vi "Open.vi"(7 "Allow multiple opens?":bool, 8 "error in (no error)":errorcluster, 10 "Channel Name":tag) -> (0 "error out":errorcluster, 3 "I2C Ref Out":T1={"myRIO Reference"={"myRIO Model"=enum."Unknown", "myRIO Hardware Reference"={"Generic FPGA Reference"=refnum, "Allow multiple opens"=FALSE}}, "I2C Channels Enum"=enum."Not Connected", "I2C Configuration"={"I2C Transfer Rate"=enum."Fast mode (400 kbps)"}})   [LabVIEW 2021, in "I2C.lvlib"]
doc: "Opens a reference to an Inter-Integrated Circuit (I2C) channel. You must open a reference before you use an I2C channel to write/read data to/from an I2C slave device."
uses:
  <vilib>/myRIO/Instrument Drivers/Onboard IO/I2C/I2C.lvlib
  <vilib>/myRIO/Instrument Drivers/Onboard IO/I2C/typedefs/I2C Reference.ctl
  <vilib>/myRIO/Common/Instrument Driver Framework/Utilities/typedefs/myRIO Generic Hardware Reference.ctl
  <vilib>/myRIO/Common/Instrument Driver Framework/Utilities/typedefs/Hardware Version Enum.ctl
  <vilib>/myRIO/Common/Instrument Driver Framework/Utilities/typedefs/myRIO v1.0 Reference.ctl
  <vilib>/myRIO/Common/Instrument Driver Framework/Utilities/typedefs/Generic FPGA Reference.ctl
  <vilib>/myRIO/Common/Instrument Driver Framework/myRIO v1.0/I2C/typedefs/I2C Channels Enum.ctl
  <vilib>/myRIO/Instrument Drivers/Onboard IO/I2C/typedefs/I2C Configuration.ctl
  <vilib>/myRIO/Instrument Drivers/Onboard IO/I2C/typedefs/I2C Transfer Rate.ctl
  <vilib>/myRIO/Common/Instrument Driver Framework/Utilities/vis/Validate Channels.vi
  <vilib>/myRIO/Common/Instrument Driver Framework/myRIO v1.0/I2C/vis/myRIO v1.0 Reserve I2C.vi
  <vilib>/myRIO/Common/Instrument Driver Framework/roboRIO v1.0/I2C/vis/roboRIO v1.0 Reserve I2C.vi
  <vilib>/myRIO/Common/Instrument Driver Framework/ELVIS III v1.0/I2C/vis/ELVIS III v1.0 Reserve I2C.vi
  <vilib>/myRIO/Common/Instrument Driver Framework/myRIO v1.0/I2C/vis/myRIO v1.0 Build MUX Configuration I2C.vi
  <vilib>/myRIO/Common/Instrument Driver Framework/myRIO v1.0/Resource Manager/vis/myRIO v1.0 Reserve Channel List.vi
  <vilib>/myRIO/Common/Instrument Driver Framework/roboRIO v1.0/Resource Manager/vis/roboRIO v1.0 Reserve Channel List.vi
  <vilib>/myRIO/Common/Instrument Driver Framework/roboRIO v1.0/I2C/vis/roboRIO v1.0 Build MUX Configuration I2C.vi
  <vilib>/myRIO/Common/Instrument Driver Framework/ELVIS III v1.0/I2C/vis/ELVIS III v1.0 Build MUX Configuration I2C.vi
  <vilib>/myRIO/Common/Instrument Driver Framework/myRIO v1.0/Resource Manager/vis/myRIO v1.0 Create Configuration List.vi
  <vilib>/myRIO/Common/Instrument Driver Framework/myRIO v1.0/Resource Manager/vis/myRIO v1.0 Reserve Channel.vi
  <vilib>/myRIO/Common/Instrument Driver Framework/myRIO v1.0/Resource Manager/vis/myRIO v1.0 Unreserve Channel.vi
  <vilib>/myRIO/Common/Instrument Driver Framework/roboRIO v1.0/Resource Manager/vis/roboRIO v1.0 Reserve Channel.vi
  <vilib>/myRIO/Common/Instrument Driver Framework/roboRIO v1.0/Resource Manager/vis/roboRIO v1.0 Unreserve Channel.vi
  <vilib>/myRIO/Common/Instrument Driver Framework/roboRIO v1.0/Resource Manager/vis/roboRIO v1.0 Create Configuration List.vi
  <vilib>/myRIO/Common/Instrument Driver Framework/ELVIS III v1.0/Resource Manager/vis/ELVIS III v1.0 Create Configuration List.vi
  <vilib>/myRIO/Common/Instrument Driver Framework/myRIO v1.0/Resource Manager/vis/myRIO v1.0 Build Mutex Name.vi
  <vilib>/myRIO/Common/Instrument Driver Framework/roboRIO v1.0/Resource Manager/vis/roboRIO v1.0 Build Mutex Name.vi
  <vilib>/Utility/VariantDataType/GetNumericInfo.vi
  <vilib>/myRIO/Common/Instrument Driver Framework/Utilities/vis/IO Manager.vi
  <vilib>/myRIO/Common/Instrument Driver Framework/Utilities/vis/Configuration Manager.vi
  <vilib>/myRIO/Common/Instrument Driver Framework/myRIO v1.0/Resource Manager/vis/myRIO v1.0 Configure IO.vi
  <vilib>/myRIO/Common/Instrument Driver Framework/myRIO v1.0/myRIO v1.0 Close.vi
  <vilib>/myRIO/Common/Instrument Driver Framework/roboRIO v1.0/Resource Manager/vis/roboRIO v1.0 Configure IO.vi
  <vilib>/myRIO/Common/Instrument Driver Framework/ELVIS III v1.0/Resource Manager/vis/ELVIS III v1.0 Reserve Channel List.vi
  <vilib>/myRIO/Common/Instrument Driver Framework/ELVIS III v1.0/Resource Manager/vis/ELVIS III v1.0 Configure IO.vi
  <vilib>/userdefined/High Color/nirio_resource_hc.ctl
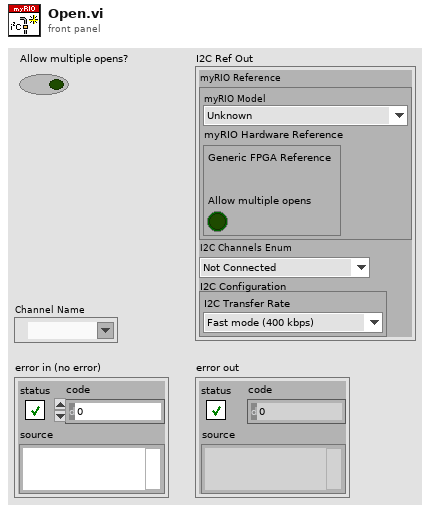
[diagram p1: front panel]
types:
  T1 = typedef "I2C.lvlib/I2C Reference.ctl" = cluster{"myRIO Reference":T2, "I2C Channels Enum":T6, "I2C Configuration":T7}
  T2 = typedef "myRIO Generic Hardware Reference.ctl" = cluster{"myRIO Model":T3, "myRIO Hardware Reference":T4}
  T3 = typedef "Hardware Version Enum.ctl" = enum16{"Unknown", "myRIO-1900", "myRIO-1950", "roboRIO", "NI ELVIS RIO CM", "ELVIS III"}
  T4 = typedef "myRIO v1.0 Reference.ctl" = cluster{"Generic FPGA Reference":T5, "Allow multiple opens":bool}
  T5 = typedef "Generic FPGA Reference.ctl" = refnum<k20>
  T6 = typedef "I2C Channels Enum.ctl" = enum16{"Not Connected", "A/I2C", "B/I2C", "I2C/I2C"}
  T7 = typedef "I2C.lvlib/I2C Configuration.ctl" = cluster{"I2C Transfer Rate":T8}
  T8 = typedef "I2C.lvlib/I2C Transfer Rate.ctl" = enum16{"Standard mode (100 kbps)", "Fast mode (400 kbps)"}
  T9 = typedef "nirio_resource_hc.ctl" = tag
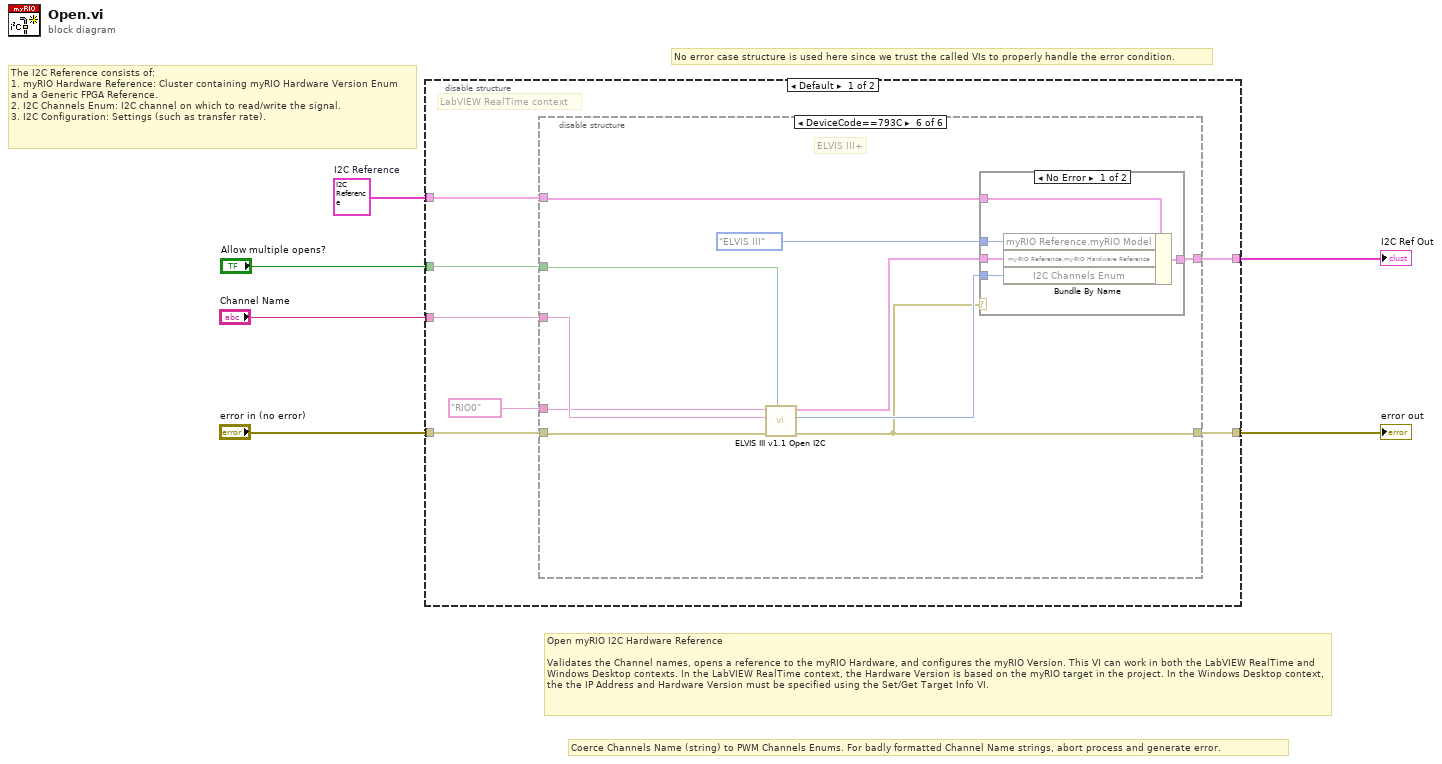
[diagram p0: block diagram]
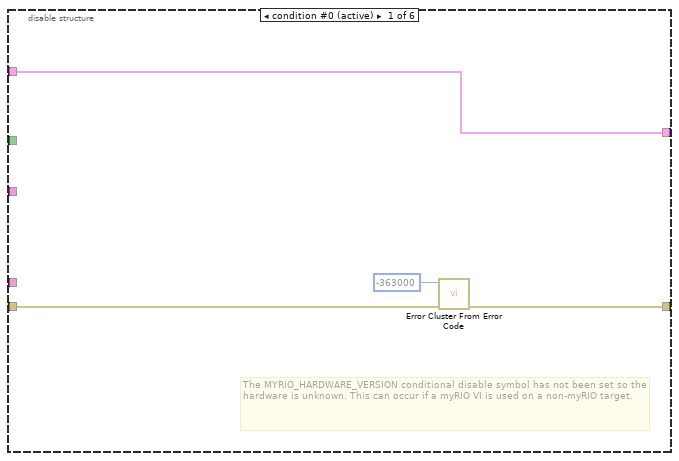
[diagram p2: hidden frame]
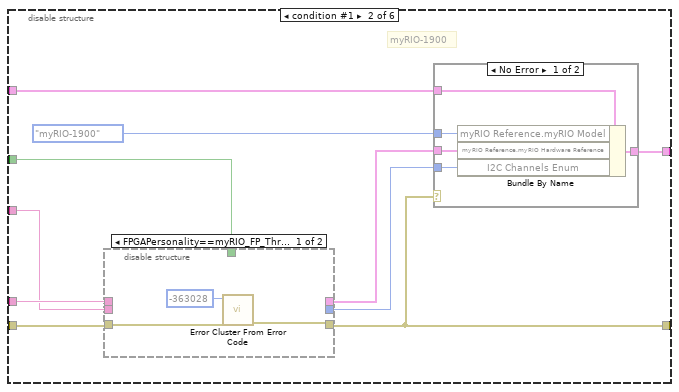
[diagram p3: hidden frame]
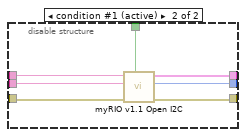
[diagram p4: hidden frame]
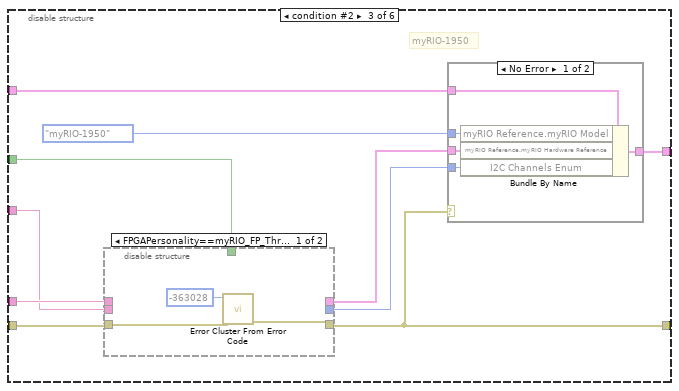
[diagram p6: hidden frame]
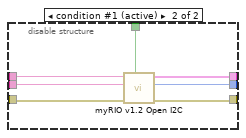
[diagram p7: hidden frame]
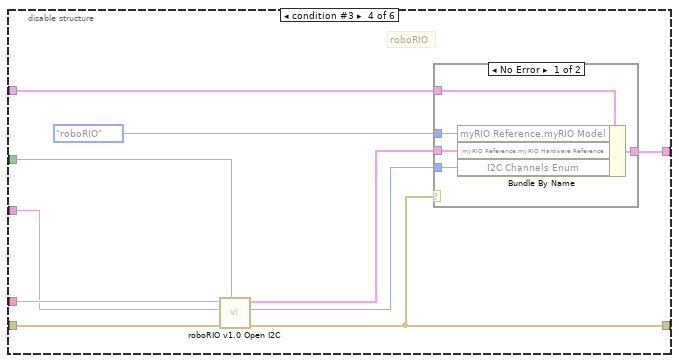
[diagram p9: hidden frame]
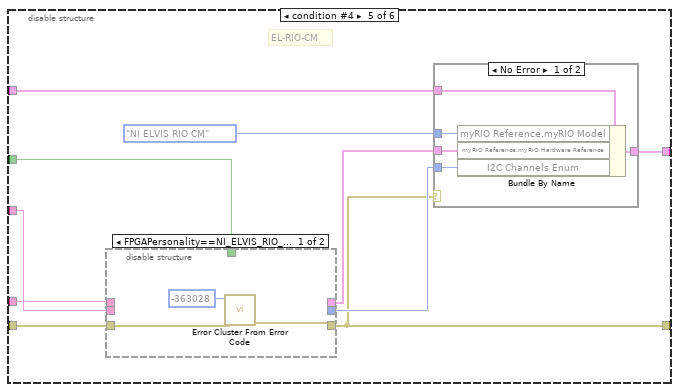
[diagram p11: hidden frame]
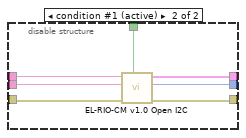
[diagram p12: hidden frame]
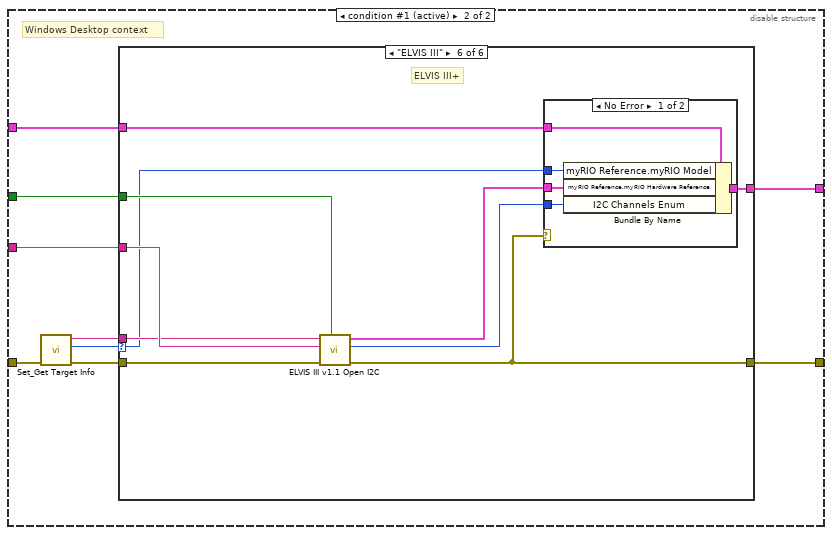
[diagram p15: hidden frame]
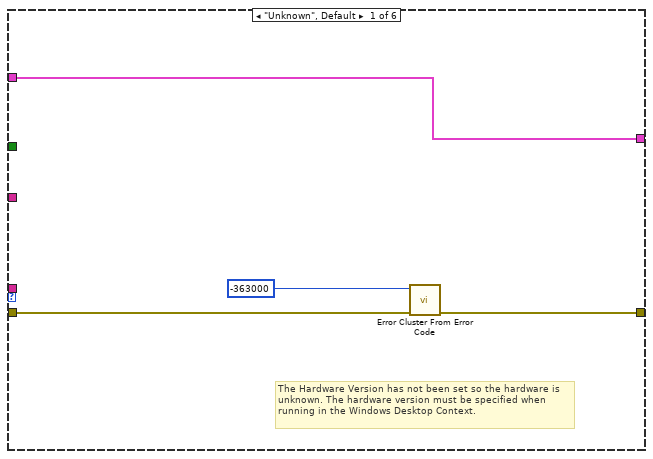
[diagram p16: hidden frame]
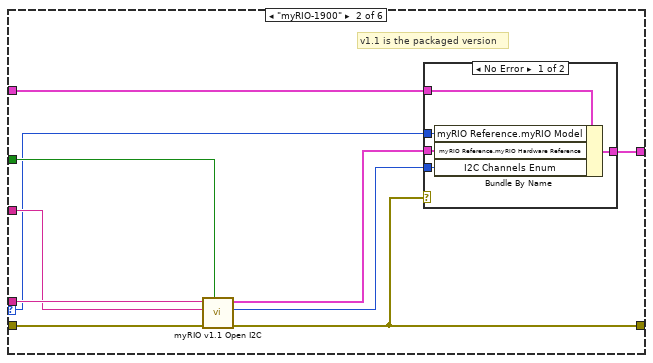
[diagram p17: hidden frame]
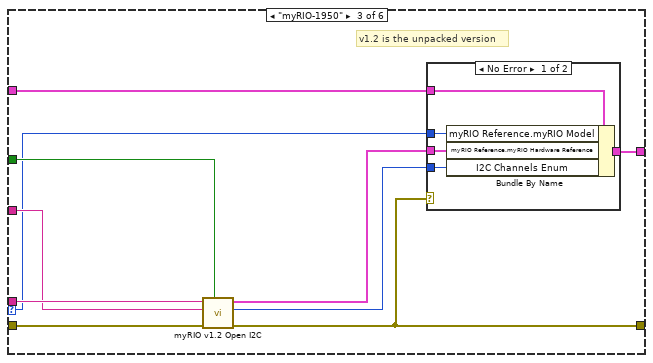
[diagram p19: hidden frame]
diagram:
  w6 = T1 {"myRIO Reference"={"myRIO Model"=enum."Unknown", "myRIO Hardware Reference"={"Generic FPGA Reference"=refnum, "Allow multiple opens"=FALSE}}, "I2C Channels Enum"=enum."Not Connected", "I2C Configuration"={"I2C Transfer Rate"=enum."Standard mode (100 kbps)"}}  # I2C Reference
  # "No error case structure is used here since we trust the called VIs to properly handle the error condition."
  # "Open myRIO I2C Hardware Reference\n\nValidates the Channel names, opens a reference to the myRIO Hardware, and configures the myRIO Version. This VI can work in both the LabVIEW RealTime and Windows Desktop contexts. In the LabVIEW RealTime context, the Hardware Version is based on the myRIO target in the project. In the Windows Desktop context, the the IP Address and Hardware Version must be specified using the Set/Get Target Info VI."
  # "The I2C Reference consists of:\n1. myRIO Hardware Reference: Cluster containing myRIO Hardware Version Enum and a Generic FPGA Reference.\n2. I2C Channels Enum: I2C channel on which to read/write the signal.\n3. I2C Configuration: Settings (such as transfer rate)."
  # "Coerce Channels Name (string) to PWM Channels Enums. For badly formatted Channel Name strings, abort process and generate error."
  n1 = disable-structure shown="Default" {
    disable-tunnel: [w13 w136] -> w4
    disable-tunnel: "error in (no error)" -> [w12 w133]
    disable-tunnel: [w11 w135] -> w3
    disable-tunnel: w6 -> [w10 w134]
    disable-tunnel: "Channel Name" -> [w8 w129]
    disable-tunnel: "Allow multiple opens?" -> [w7 w128]
    frame condition #0 {
      # "LabVIEW RealTime context"
      n2 = disable-structure shown="DeviceCode==793C" {
        disable-tunnel: [w16 w18 w44 w70 w87 w113] -> w13
        disable-tunnel: [w14 w24 w50 w76 w94 w112] -> w11
        disable-tunnel: w12 -> [w15 w25 w51 w77 w92 w114]
        disable-tunnel: w10 -> [w14 w23 w49 w75 w93 w118]
        disable-tunnel: T9 "RIO0" ("resource name") -> [_ w22 w48 w74 w90 w115]
        disable-tunnel: w8 -> [_ w21 w47 w73 w91 w116]
        disable-tunnel: w7 -> [_ w19 w45 w71 w86 w117]
        frame condition #0 (active) {
          # "The MYRIO_HARDWARE_VERSION conditional disable symbol has not been set so the hardware is unknown. This can occur if a myRIO VI is used on a non-myRIO target."
          n3 = call <vilib>:"Error Cluster From Error Code.vi"("error in (no error)"=w15, "error code (0)"=-363000) -> ("error out"=w16:errorcluster)  [unwired: 7 in]
        }
        frame condition #1 {
          # "myRIO-1900"
          n4 = disable-structure shown="FPGAPersonality==myRIO_FP_Throughput" {
            disable-tunnel: [_ w37] -> w26
            disable-tunnel: w25 -> [w29 w36]
            disable-tunnel: w22 -> [_ w35]
            disable-tunnel: w21 -> [_ w34]
            disable-tunnel: [_ w33] -> w20
            disable-tunnel: w19 -> [_ w32]
            disable-tunnel: [w28 w31] -> w18
            frame condition #0 {
              n5 = call <vilib>:"Error Cluster From Error Code.vi"("error in (no error)"=w29, "error code (0)"=-363028) -> ("error out"=w28:errorcluster)  [unwired: 7 in]
            }
            frame condition #1 (active) {
              n6 = call <vilib>:"myRIO v1.1 Open I2C.vi"("Allow multiple opens?"=w32, "error in (no error)"=w36, "Channel Name"=w34, "Resource name"=w35) -> ("error out"=w31:errorcluster, "I2C Channel"=w33:T6, "myRIO Ref Out"=w37:T4)  [unwired: 5 in]
            }
          }
          n7 = case shown="No Error" w18 {
            tunnel: Hardware_Version_Enum."myRIO-1900" ("Hardware Version") -> [w42 _]
            tunnel: w26 -> [w41 _]
            tunnel: [w40 w43] -> w24
            tunnel: w23 -> [w39 w43]
            tunnel: w20 -> [w38 _]
            frame No Error {
              n8 = Bundle By Name(cluster=w39, "myRIO Reference.myRIO Model"=w42, "myRIO Reference.myRIO Hardware Reference"=w41, "I2C Channels Enum"=w38) -> (w40:T1)
            }
            frame Error {
            }
          }
        }
        frame condition #2 {
          # "myRIO-1950"
          n9 = disable-structure shown="FPGAPersonality==myRIO_FP_Throughput" {
            disable-tunnel: [_ w63] -> w52
            disable-tunnel: w51 -> [w55 w62]
            disable-tunnel: w48 -> [_ w61]
            disable-tunnel: w47 -> [_ w60]
            disable-tunnel: [_ w59] -> w46
            disable-tunnel: w45 -> [_ w58]
            disable-tunnel: [w54 w57] -> w44
            frame condition #0 {
              n10 = call <vilib>:"Error Cluster From Error Code.vi"("error in (no error)"=w55, "error code (0)"=-363028) -> ("error out"=w54:errorcluster)  [unwired: 7 in]
            }
            frame condition #1 (active) {
              n11 = call <vilib>:"myRIO v1.2 Open I2C.vi"("Allow multiple opens?"=w58, "error in (no error)"=w62, "Channel Name"=w60, "Resource name"=w61) -> ("error out"=w57:errorcluster, "I2C Channel"=w59:T6, "myRIO Ref Out"=w63:T4)  [unwired: 5 in]
            }
          }
          n12 = case shown="No Error" w44 {
            tunnel: Hardware_Version_Enum."myRIO-1950" ("Hardware Version") -> [w68 _]
            tunnel: w52 -> [w67 _]
            tunnel: [w66 w69] -> w50
            tunnel: w49 -> [w65 w69]
            tunnel: w46 -> [w64 _]
            frame No Error {
              n13 = Bundle By Name(cluster=w65, "myRIO Reference.myRIO Model"=w68, "myRIO Reference.myRIO Hardware Reference"=w67, "I2C Channels Enum"=w64) -> (w66:T1)
            }
            frame Error {
            }
          }
        }
        frame condition #3 {
          # "roboRIO"
          n14 = call <vilib>:"roboRIO v1.0 Open I2C.vi"("Allow multiple opens?"=w71, "error in (no error)"=w77, "Channel Name"=w73, "Resource name"=w74) -> ("error out"=w70:errorcluster, "I2C Channel"=w72:T6, "myRIO Ref Out"=w78:T4)  [unwired: 5 in]
          n15 = case shown="No Error" w70 {
            tunnel: Hardware_Version_Enum."roboRIO" ("Hardware Version") -> [w84 _]
            tunnel: w78 -> [w83 _]
            tunnel: [w82 w85] -> w76
            tunnel: w75 -> [w81 w85]
            tunnel: w72 -> [w80 _]
            frame No Error {
              n16 = Bundle By Name(cluster=w81, "myRIO Reference.myRIO Model"=w84, "myRIO Reference.myRIO Hardware Reference"=w83, "I2C Channels Enum"=w80) -> (w82:T1)
            }
            frame Error {
            }
          }
        }
        frame condition #4 {
          # "EL-RIO-CM"
          n17 = disable-structure shown="FPGAPersonality==NI_ELVIS_RIO_CM_FP_Throughput" {
            disable-tunnel: [_ w105] -> w89
            disable-tunnel: w92 -> [w97 w100]
            disable-tunnel: w90 -> [_ w102]
            disable-tunnel: w91 -> [_ w101]
            disable-tunnel: [_ w104] -> w88
            disable-tunnel: w86 -> [_ w99]
            disable-tunnel: [w96 w103] -> w87
            frame condition #0 {
              n18 = call <vilib>:"Error Cluster From Error Code.vi"("error in (no error)"=w97, "error code (0)"=-363028) -> ("error out"=w96:errorcluster)  [unwired: 7 in]
            }
            frame condition #1 (active) {
              n19 = call <vilib>:"EL-RIO-CM v1.0 Open I2C.vi"("Allow multiple opens?"=w99, "error in (no error)"=w100, "Channel Name"=w101, "Resource name"=w102) -> ("error out"=w103:errorcluster, "I2C Channel"=w104:T6, "myRIO Ref Out"=w105:T4)  [unwired: 5 in]
            }
          }
          n20 = case shown="No Error" w87 {
            tunnel: Hardware_Version_Enum."NI ELVIS RIO CM" ("Hardware Version") -> [w110 _]
            tunnel: w89 -> [w109 _]
            tunnel: [w108 w111] -> w94
            tunnel: w93 -> [w107 w111]
            tunnel: w88 -> [w106 _]
            frame No Error {
              n21 = Bundle By Name(cluster=w107, "myRIO Reference.myRIO Model"=w110, "myRIO Reference.myRIO Hardware Reference"=w109, "I2C Channels Enum"=w106) -> (w108:T1)
            }
            frame Error {
            }
          }
        }
        frame condition #5 {
          # "ELVIS III+"
          n22 = call <vilib>:"ELVIS III v1.1 Open I2C.vi"("Allow multiple opens?"=w117, "error in (no error)"=w114, "Channel Name"=w116, "Resource name"=w115) -> ("error out"=w113:errorcluster, "I2C Channel"=w119:T6, "myRIO Ref Out"=w120:T4)  [unwired: 5 in]
          n23 = case shown="No Error" w113 {
            tunnel: Hardware_Version_Enum."ELVIS III" ("Hardware Version") -> [w126 _]
            tunnel: w120 -> [w125 _]
            tunnel: [w124 w127] -> w112
            tunnel: w118 -> [w123 w127]
            tunnel: w119 -> [w122 _]
            frame No Error {
              n24 = Bundle By Name(cluster=w123, "myRIO Reference.myRIO Model"=w126, "myRIO Reference.myRIO Hardware Reference"=w125, "I2C Channels Enum"=w122) -> (w124:T1)
            }
            frame Error {
            }
          }
        }
      }
    }
    frame condition #1 (active) {
      # "Windows Desktop context"
      n25 = call <vilib>:"Set_Get Target Info.vi"("error in (no error)"=w133) -> ("error out"=w132:errorcluster, "Hardware Version"=w131:T3, "IP Address"=w130:string)  [unwired: 8 in]
      n26 = case shown="\"ELVIS III\"" w131 {
        selector: w131 -> [_ w141 w157 w173 w189 w208]
        tunnel: [w139 w142 w158 w174 w190 w206] -> w136
        tunnel: w132 -> [w138 w147 w163 w179 w195 w207]
        tunnel: [w137 w149 w165 w181 w197 w205] -> w135
        tunnel: w134 -> [w137 w148 w164 w180 w196 w212]
        tunnel: w130 -> [_ w146 w162 w178 w194 w209]
        tunnel: w129 -> [_ w145 w161 w177 w193 w210]
        tunnel: w128 -> [_ w143 w159 w175 w191 w211]
        frame "Unknown", Default {
          # "The Hardware Version has not been set so the hardware is unknown. The hardware version must be specified when running in the Windows Desktop Context."
          n27 = call <vilib>:"Error Cluster From Error Code.vi"("error in (no error)"=w138, "error code (0)"=-363000) -> ("error out"=w139:errorcluster)  [unwired: 7 in]
        }
        frame "myRIO-1900" {
          # "v1.1 is the packaged version"
          n28 = call <vilib>:"myRIO v1.1 Open I2C.vi"("Allow multiple opens?"=w143, "error in (no error)"=w147, "Channel Name"=w145, "Resource name"=w146) -> ("error out"=w142:errorcluster, "I2C Channel"=w144:T6, "myRIO Ref Out"=w150:T4)  [unwired: 5 in]
          n29 = case shown="No Error" w142 {
            tunnel: w141 -> [w155 _]
            tunnel: w150 -> [w154 _]
            tunnel: [w153 w156] -> w149
            tunnel: w148 -> [w152 w156]
            tunnel: w144 -> [w151 _]
            frame No Error {
              n30 = Bundle By Name(cluster=w152, "myRIO Reference.myRIO Model"=w155, "myRIO Reference.myRIO Hardware Reference"=w154, "I2C Channels Enum"=w151) -> (w153:T1)
            }
            frame Error {
            }
          }
        }
        frame "myRIO-1950" {
          # "v1.2 is the unpacked version"
          n31 = call <vilib>:"myRIO v1.2 Open I2C.vi"("Allow multiple opens?"=w159, "error in (no error)"=w163, "Channel Name"=w161, "Resource name"=w162) -> ("error out"=w158:errorcluster, "I2C Channel"=w160:T6, "myRIO Ref Out"=w166:T4)  [unwired: 5 in]
          n32 = case shown="No Error" w158 {
            tunnel: w157 -> [w171 _]
            tunnel: w166 -> [w170 _]
            tunnel: [w169 w172] -> w165
            tunnel: w164 -> [w168 w172]
            tunnel: w160 -> [w167 _]
            frame No Error {
              n33 = Bundle By Name(cluster=w168, "myRIO Reference.myRIO Model"=w171, "myRIO Reference.myRIO Hardware Reference"=w170, "I2C Channels Enum"=w167) -> (w169:T1)
            }
            frame Error {
            }
          }
        }
        frame "roboRIO" {
          # "v1.2 is the unpacked version"
          n34 = call <vilib>:"roboRIO v1.0 Open I2C.vi"("Allow multiple opens?"=w175, "error in (no error)"=w179, "Channel Name"=w177, "Resource name"=w178) -> ("error out"=w174:errorcluster, "I2C Channel"=w176:T6, "myRIO Ref Out"=w182:T4)  [unwired: 5 in]
          n35 = case shown="No Error" w174 {
            tunnel: w173 -> [w187 _]
            tunnel: w182 -> [w186 _]
            tunnel: [w185 w188] -> w181
            tunnel: w180 -> [w184 w188]
            tunnel: w176 -> [w183 _]
            frame No Error {
              n36 = Bundle By Name(cluster=w184, "myRIO Reference.myRIO Model"=w187, "myRIO Reference.myRIO Hardware Reference"=w186, "I2C Channels Enum"=w183) -> (w185:T1)
            }
            frame Error {
            }
          }
        }
        frame "NI ELVIS RIO CM" {
          # "EL-RIO-CM"
          n37 = call <vilib>:"EL-RIO-CM v1.0 Open I2C.vi"("Allow multiple opens?"=w191, "error in (no error)"=w195, "Channel Name"=w193, "Resource name"=w194) -> ("error out"=w190:errorcluster, "I2C Channel"=w192:T6, "myRIO Ref Out"=w198:T4)  [unwired: 5 in]
          n38 = case shown="No Error" w190 {
            tunnel: w189 -> [w203 _]
            tunnel: w198 -> [w202 _]
            tunnel: [w201 w204] -> w197
            tunnel: w196 -> [w200 w204]
            tunnel: w192 -> [w199 _]
            frame No Error {
              n39 = Bundle By Name(cluster=w200, "myRIO Reference.myRIO Model"=w203, "myRIO Reference.myRIO Hardware Reference"=w202, "I2C Channels Enum"=w199) -> (w201:T1)
            }
            frame Error {
            }
          }
        }
        frame "ELVIS III" {
          # "ELVIS III+"
          n40 = call <vilib>:"ELVIS III v1.1 Open I2C.vi"("Allow multiple opens?"=w211, "error in (no error)"=w207, "Channel Name"=w210, "Resource name"=w209) -> ("error out"=w206:errorcluster, "I2C Channel"=w213:T6, "myRIO Ref Out"=w214:T4)  [unwired: 5 in]
          n41 = case shown="No Error" w206 {
            tunnel: w208 -> [w219 _]
            tunnel: w214 -> [w218 _]
            tunnel: [w217 w220] -> w205
            tunnel: w212 -> [w216 w220]
            tunnel: w213 -> [w215 _]
            frame No Error {
              n42 = Bundle By Name(cluster=w216, "myRIO Reference.myRIO Model"=w219, "myRIO Reference.myRIO Hardware Reference"=w218, "I2C Channels Enum"=w215) -> (w217:T1)
            }
            frame Error {
            }
          }
        }
      }
    }
  }
  "I2C Ref Out" <- w3
  "error out" <- w4
